vi "Set_Reset_Ch.vi"(0 "device name":tag="Dev0", 1 "SetReset":bool=TRUE, 7 "Ch":T1(ring), 11 "error in":errorcluster) -> (8 "error out":errorcluster)   [LabVIEW 2017]
panel:
  out "error out 2":errorcluster
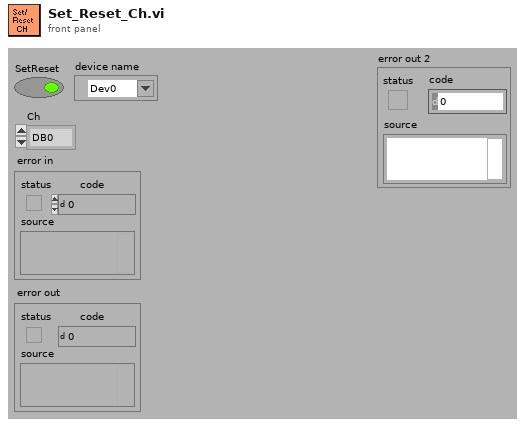
[diagram p1: front panel]
types:
  T1 = enum16{"DB0", "DB1", "DB2", "DB3", "DB4", "DB5", "DB6", "DB7", "DB8", "DB9", "DB10", "DB11", "A0", "A1", "RW", "LDAC", "ADMAIN1", "ADMAIN2", "ADMAIN3", "G1", "CS", "CLR", "P0", "P1"}
  T2 = enum16{"Reset", "Update U1", "Update U2", "Update U3", "Read all"}
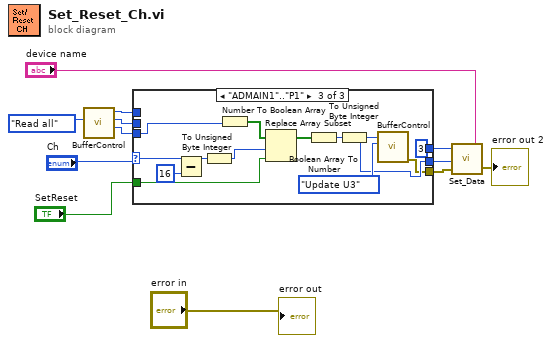
[diagram p0: block diagram]
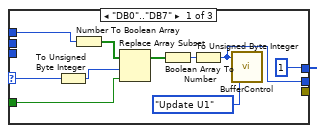
[diagram p2: hidden frame]
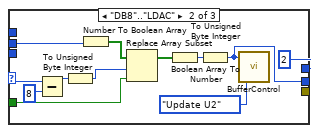
[diagram p3: hidden frame]
diagram:
  n1 = call "BufferControl.vi"("Enum"=T2."Read all") -> ("U3BuffRead"=w8:u8, "U2BuffRead"=w9:u8, "U1BuffRead"=w10:u8)  [unwired: 3 in, 1 out]
  n2 = case shown="\"ADMAIN1\"..\"P1\"" "Ch" {
    selector: "Ch" -> [w20 w26 w39]
    tunnel: w10 -> [w22 _ _]
    tunnel: w9 -> [_ w28 _]
    tunnel: w8 -> [_ _ w41]
    tunnel: "SetReset" -> [w19 w29 w40]
    tunnel: [w13 w23 w37] -> w5
    tunnel: [u8 1 ("Ch") u8 2 ("Ch") u8 3 ("Ch")] -> w4
    tunnel: [_ _ w35] -> w2
    frame "DB0".."DB7" {
      n3 = To Unsigned Byte Integer(number=w20) -> (unsigned 8bit integer=w18:u8)
      n4 = Number To Boolean Array(number=w22) -> (Boolean array=w21:bool[])
      n5 = Replace Array Subset(array=w21, new element=w19, index=w18) -> (w17:bool[])
      n6 = Boolean Array To Number(Boolean array=w17) -> (number=w15:u32)
      n7 = To Unsigned Byte Integer(number=w15) -> (unsigned 8bit integer=w13:u8)
      n8 = call "BufferControl.vi"("Enum"=T2."Update U1", "Data"=w13) -> ()  [unwired: 2 in, 4 out]
    }
    frame "DB8".."LDAC" {
      n9 = Subtract(x=w26, y=8) -> (x-y=w27:i32)
      n10 = To Unsigned Byte Integer(number=w27) -> (unsigned 8bit integer=w33:u8)
      n11 = Number To Boolean Array(number=w28) -> (Boolean array=w34:bool[])
      n12 = Replace Array Subset(array=w34, new element=w29, index=w33) -> (w32:bool[])
      n13 = Boolean Array To Number(Boolean array=w32) -> (number=w30:u32)
      n14 = To Unsigned Byte Integer(number=w30) -> (unsigned 8bit integer=w23:u8)
      n15 = call "BufferControl.vi"("Enum"=T2."Update U2", "Data"=w23) -> ()  [unwired: 2 in, 4 out]
    }
    frame "ADMAIN1".."P1" {
      n16 = Subtract(x=w39, y=16) -> (x-y=w42:i32)
      n17 = To Unsigned Byte Integer(number=w42) -> (unsigned 8bit integer=w46:u8)
      n18 = Number To Boolean Array(number=w41) -> (Boolean array=w47:bool[])
      n19 = Replace Array Subset(array=w47, new element=w40, index=w46) -> (w45:bool[])
      n20 = Boolean Array To Number(Boolean array=w45) -> (number=w43:u32)
      n21 = To Unsigned Byte Integer(number=w43) -> (unsigned 8bit integer=w37:u8)
      n22 = call "BufferControl.vi"("Enum"=T2."Update U3", "Data"=w37) -> ("error out"=w35:errorcluster)  [unwired: 2 in, 3 out]
    }
  }
  n23 = call "Set_Data.vi"("device name"="device name", "error in"=w2, "Data"=w5, "Ch"=w4) -> ("error out"=→"error out 2":errorcluster)
  "error out" <- "error in"
